vi "Add.vi"(11 "SimpleAdder in":refnum<class "SimpleAdder.lvclass">) -> (3 "SimpleAdder out":refnum<class "SimpleAdder.lvclass">)   [LabVIEW 2012, in "SimpleAdder.lvclass"]
uses:
  SimpleAdder.lvclass
  SimpleAdder.lvclass/SimpleAdder.ctl
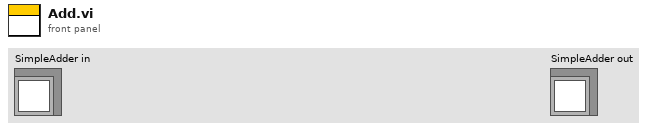
[diagram p1: front panel]
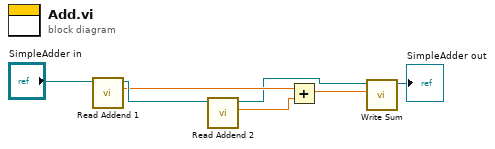
[diagram p0: block diagram]
diagram:
  n1 = call "Read Addend 1.vi"("SimpleAdder in"="SimpleAdder in") -> ("Addend 1"=w4:dbl, "SimpleAdder out"=w6:refnum<class "SimpleAdder.lvclass">)  [unwired: 8 in, 1 out]
  n2 = call "Read Addend 2.vi"("SimpleAdder in"=w6) -> ("Addend 2"=w5:dbl, "SimpleAdder out"=w3:refnum<class "SimpleAdder.lvclass">)  [unwired: 8 in, 1 out]
  n3 = Add(x=w4, y=w5) -> (x+y=w2:dbl)
  n4 = call "Write Sum.vi"("Sum"=w2, "SimpleAdder in"=w3) -> ("SimpleAdder out"=→"SimpleAdder out":refnum<class "SimpleAdder.lvclass">)  [unwired: 8 in, 1 out]
